vi "sub_ofdm_delayed_mult_CFO_sync.vi"(8 "CP length":i32=64, 9 "FFT size":i32=256, 11 "time samples":cdb[](array[numeric])) -> (0 "last index":i32, 3 "corrected OFDM symbol":cdb[][](array[numeric]))   [LabVIEW 2014]
uses:
  <vilib>/Analysis/1siggen.llb/Ramp Pattern by Samples.vi
  <vilib>/Analysis/NI_AALBase.lvlib
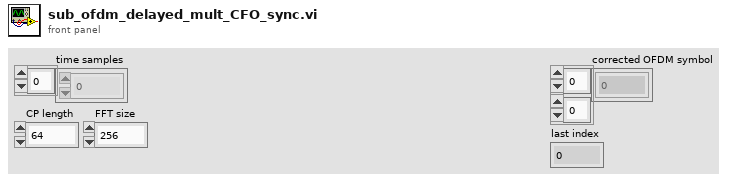
[diagram p1: front panel]
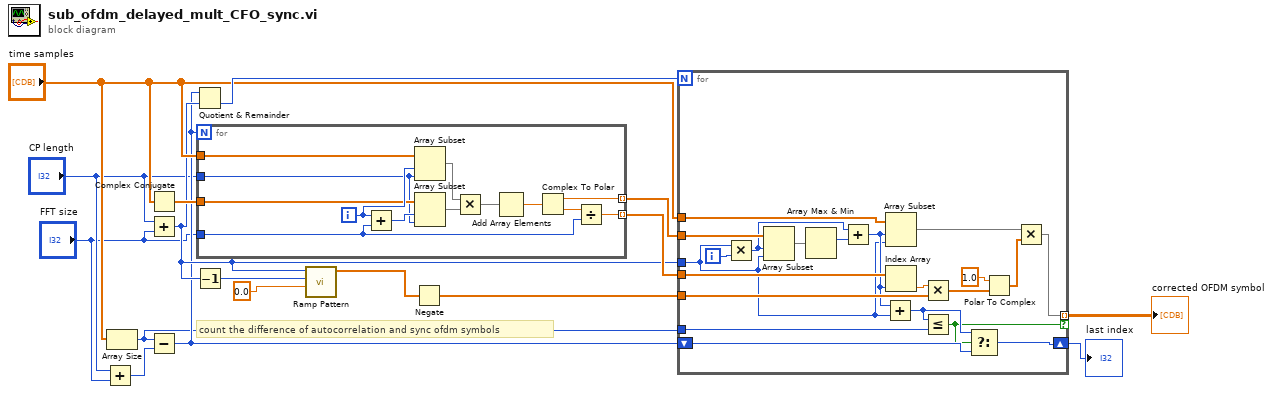
[diagram p0: block diagram]
diagram:
  # "count the difference of autocorrelation and sync ofdm symbols"
  n1 = Add(x="CP length", y="FFT size") -> (x+y=w2:i32)
  n2 = Array Size(array="time samples") -> (size(s)=w1:i32)
  n3 = Complex Conjugate(1:"time samples") -> (0:w17:cdb[])
  n4 = Add(x="CP length", y="FFT size") -> (x+y=w13:i32)
  n5 = Subtract(x=w1, y=w2) -> (x-y=w5:i32)
  n6 = Quotient & Remainder(x=w5, y=w13) -> (floor(x/y)=w15:i32)  [unwired: 1 out]
  n7 = Decrement(x=w13) -> (x-1=w12:i32)
  n8 = for {
    N: w5 -> [_]
    tunnel: "time samples" -> [w30]
    tunnel: w17 -> [w28]
    tunnel: "FFT size" -> [w18]
    tunnel: [w22] -> w16 mode=indexing
    tunnel: [w20] -> w6 mode=indexing
    tunnel: "CP length" -> [w19]
    i -> [w29]
    n9 = Add(x=w29, y=w18) -> (x+y=w27:i32)
    n10 = Array Subset(array=w30, index=w29, length=w19) -> (w25:cdb[])
    n11 = Array Subset(array=w28, index=w27, length=w19) -> (w26:cdb[])
    n12 = Multiply(x=w25, y=w26) -> (x*y=w24:cdb[])
    n13 = Add Array Elements(numeric array=w24) -> (sum=w21:cdb)
    n14 = Complex To Polar(r * e^(i*theta)=w21) -> (r=w20:dbl, theta=w23:dbl)
    n15 = Divide(x=w23, y=w18) -> (x/y=w22:dbl)
  }
  n16 = call-poly <vilib>:"Ramp Pattern.vi"("start"=0.0, "end"=w12, "samples"=w13) -> ("Ramp Pattern"=w9:dbl[])  [unwired: 7 in, 1 out]
  n17 = Negate(x=w9) -> (-x=w8:dbl[])
  n18 = for {
    N: w15 -> [_]
    tunnel: w6 -> [w51]
    tunnel: w16 -> [w45]
    tunnel: w13 -> [w37]
    tunnel: "time samples" -> [w48]
    tunnel: w8 -> [w43]
    tunnel: [w40] -> w10 mode=indexing if=w31
    shift-right: [w34] -> w7
    shift-left: w5 -> [w35]
    tunnel: w1 -> [w32]
    i -> [w50]
    n19 = Multiply(x=w37, y=w50) -> (x*y=w47:i32)
    n20 = Array Subset(array=w51, index=w47, length=w37) -> (w49:dbl[])
    n21 = Array Max & Min(array=w49) -> (max index (indices)=w46:i32)  [unwired: 3 out]
    n22 = Add(x=w47, y=w46) -> (x+y=w38:i32)
    n23 = Add(x=w38, y=w37) -> (x+y=w33:i32)
    n24 = Array Subset(array=w48, index=w38, length=w37) -> (w36:cdb[])
    n25 = Index Array(array=w45, index=w38) -> (element=w39:dbl)
    n26 = Multiply(x=w39, y=w43) -> (x*y=w42:dbl[])
    n27 = Less Or Equal?(x=w33, y=w32) -> (x <= y?=w31:bool)
    n28 = Select(t=w33, s=w31, f=w35) -> (s? t:f=w34:i32)
    n29 = Polar To Complex(1:w42, 2:1.0) -> (0:w41:cdb[])
    n30 = Multiply(x=w36, y=w41) -> (x*y=w40:cdb[])
  }
  "corrected OFDM symbol" <- w10
  "last index" <- w7
